vi "Dynamic Call VI.vi"(6 "自动销毁引用":bool, 8 "error in":errorcluster caption="错误输入", 9 "CtrlValue":variant, 10 "CtrlName":string, 11 "Vi Path":path) -> (0 "错误输出":errorcluster, 3 "vi reference":refnum<vi>)   [LabVIEW 2016, in "PanelDataNode.lvclass"]
uses:
  PanelDataNode.lvclass
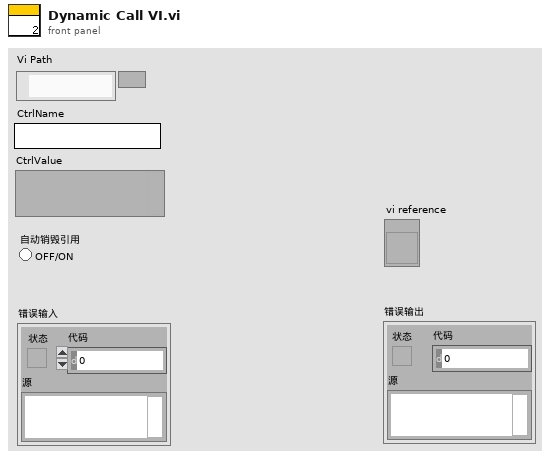
[diagram p1: front panel]
types:
  T1 = enum32{"Bad", "Idle", "Run top level", "Running"}
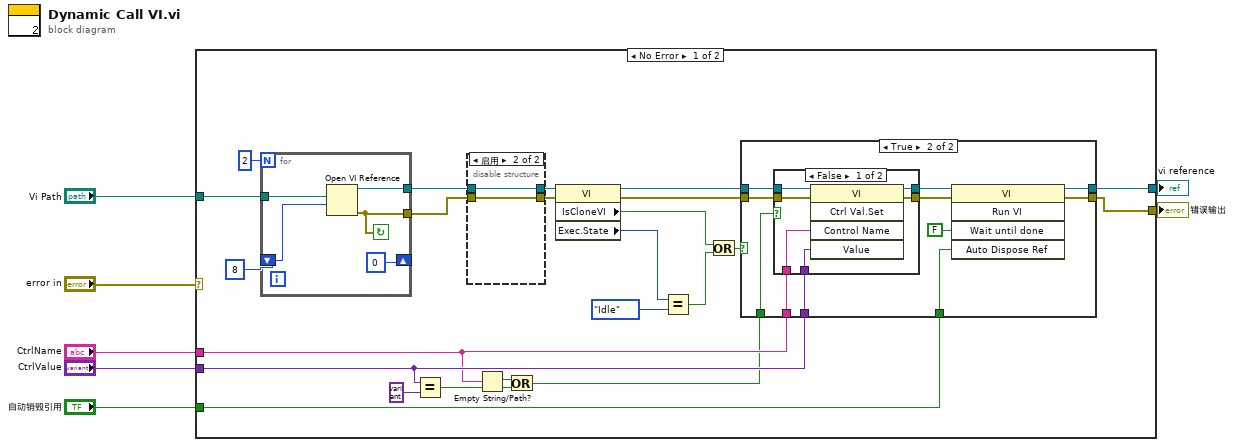
[diagram p0: block diagram]
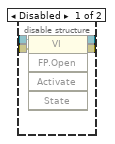
[diagram p2: hidden frame]
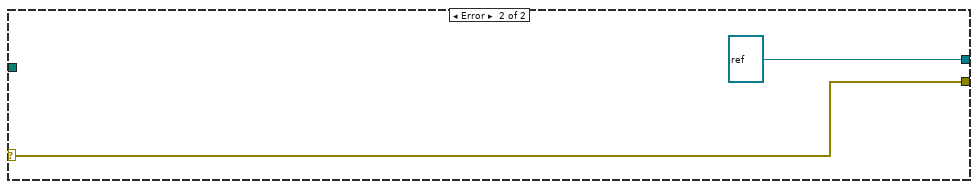
[diagram p5: hidden frame]
diagram:
  n1 = case shown="No Error" "error in" {
    selector: "error in" -> [_ w63]
    tunnel: "Vi Path" -> [w30 _]
    tunnel: [w20 refnum<vi> refnum ("vi reference")] -> w6
    tunnel: [w19 w63] -> w5
    tunnel: "自动销毁引用" -> [w18 _]
    tunnel: "CtrlName" -> [w11 _]
    tunnel: "CtrlValue" -> [w13 _]
    frame No Error {
      n2 = for {
        N: 2 -> [_]
        tunnel: w30 -> [w41]
        shift-right: [0 ("选项")] -> _
        shift-left: 8 ("选项") -> [w40]
        tunnel: [w38] -> w15
        tunnel: [w37] -> w17
        stop <- w38 continue-if-true
        n3 = Open VI Reference(vi path=w41, options=w40) -> (vi reference=w37:refnum<vi>, error out=w38:errorcluster)  [unwired: 4 in]
      }
      n4 = Equal?(x=w13, y=variant) -> (x = y?=w9:bool)
      n5 = disable-structure shown="启用" {
        disable-tunnel: w17 -> [w34 w36]
        disable-tunnel: [w33 w36] -> w16
        disable-tunnel: w15 -> [w32 w35]
        disable-tunnel: [w31 w35] -> w14
        frame Disabled {
          n6 = invoke class="VI" method="FP.Open"(reference=w34, error in=w32) -> (reference out=w33:refnum<vi>, error out=w31:errorcluster)  [unwired: 3 in, 3 out]
        }
        frame Enabled {
        }
      }
      n7 = Empty String/Path?(string/path=w11) -> (empty?=w10:bool)
      n8 = Or(x=w10, y=w9) -> (x .or. y?=w8:bool)
      n9 = property class="VI"(reference=w16, error in=w14) -> (reference out=w29:refnum<vi>, error out=w28:errorcluster, "IsCloneVI"=w23:bool, "Exec.State"=w24:T1)
      n10 = Equal?(x=w24, y=T1."Idle") -> (x = y?=w22:bool)
      n11 = Or(x=w23, y=w22) -> (x .or. y?=w21:bool)
      n12 = case shown="True" w21 {
        tunnel: w29 -> [w43 w50]
        tunnel: [w43 w54] -> w20
        tunnel: w28 -> [w42 w48]
        tunnel: [w42 w53] -> w19
        tunnel: w18 -> [_ w51]
        tunnel: w11 -> [_ w46]
        tunnel: w13 -> [_ w45]
        tunnel: w8 -> [_ w44]
        frame False {
        }
        frame True {
          n13 = case shown="False" w44 {
            tunnel: w50 -> [w60 w62]
            tunnel: [w59 w62] -> w49
            tunnel: w48 -> [w58 w61]
            tunnel: [w57 w61] -> w47
            tunnel: w46 -> [w56 _]
            tunnel: w45 -> [w55 _]
            frame False {
              n14 = invoke class="VI" method="Ctrl Val.Set"(reference=w60, error in=w58, "Control Name"=w56, "Value"=w55) -> (reference out=w59:refnum<vi>, error out=w57:errorcluster)  [unwired: 1 in, 3 out]
            }
            frame True {
            }
          }
          n15 = invoke class="VI" method="Run VI"(reference=w49, error in=w47, "Wait until done"=FALSE ("结束前等待"), "Auto Dispose Ref"=w51) -> (reference out=w54:refnum<vi>, error out=w53:errorcluster)  [unwired: 1 in, 3 out]
        }
      }
    }
    frame Error {
    }
  }
  "vi reference" <- w6
  "错误输出" <- w5
